vi "FITSWriteHeaderData.vi"(0 "CFitsIO in":refnum<class "CFitsIO.lvclass">, 1 "ref":u64, 5 "datatype":i32, 7 "keyname":string, 9 "value":string, 11 "error in (no error)":errorcluster, 12 "comment":string) -> (4 "CFitsIO out":refnum<class "CFitsIO.lvclass">, 15 "error out":errorcluster)   [LabVIEW 2016, in "CFitsIO.lvclass"]
uses:
  CFitsIO.lvclass
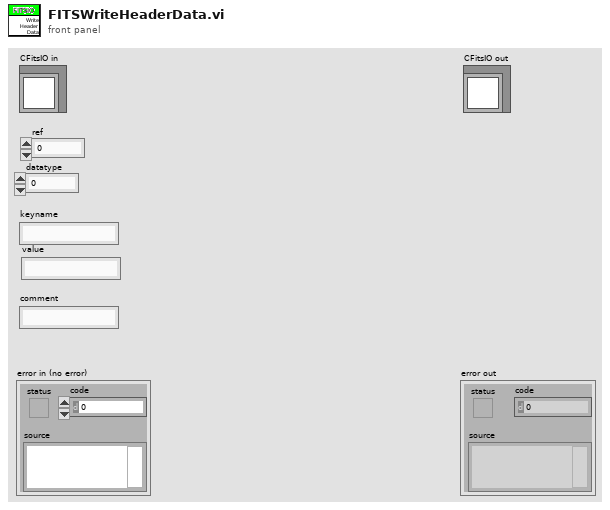
[diagram p1: front panel]
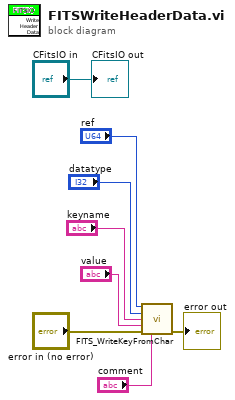
[diagram p0: block diagram]
diagram:
  n1 = call "FITS_WriteKeyFromChar.vi"("ref"="ref", "datatype"="datatype", "keyname"="keyname", "value"="value", "error in (no error)"="error in (no error)", "comment"="comment") -> ("error out"=→"error out":errorcluster)  [unwired: 5 in, 4 out]
  "CFitsIO out" <- "CFitsIO in"
